vi "导出监测.vi"(4 "路径":path, 5 "错误常量":errorcluster caption="错误输入", 6 "报警信息":string[][](array[string]), 7 "计算数据":dbl[][](array[numeric]), 8 "监测名":string) -> (0 "错误常量 2":errorcluster caption="错误输出")   [LabVIEW 2018]
uses:
  <vilib>/Utility/file.llb/Write Delimited Spreadsheet (string).vi
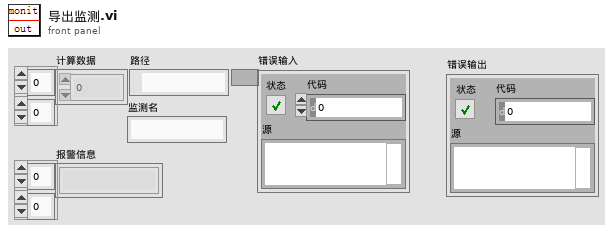
[diagram p1: front panel]
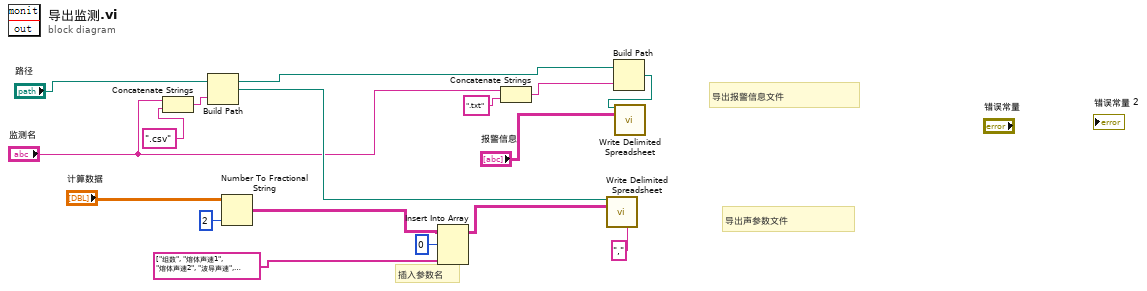
[diagram p0: block diagram]
diagram:
  # "导出声参数文件"
  # "导出报警信息文件"
  # "插入参数名"
  n1 = Concatenate Strings("监测名", ".csv" ("名称或相对路径")) -> (w14:string)
  n2 = Build Path(base path="路径", name or relative path=w14) -> (appended path=w16:path)
  n3 = Number To Fractional String(number="计算数据", precision (6)=i16 2 ("精度(6)")) -> (F-format string=w9:string[][])  [unwired: 2 in]
  n4 = Insert Into Array(array=w9, index (row)=0 ("索引 (行)"), new element=string[] ["组数", "熔体声速1", "熔体声速2", "波导声速", "声衰减系数", "声参量1  ", "声参量2  ", "x1", "x2     ", "x3", "x4       ", "y1", "y2", "y3", "y4"] ("新元素/子数组")) -> (w1:string[][])  [unwired: 1 in]
  n5 = Concatenate Strings("监测名", ".txt" ("字符串")) -> (w12:string)
  n6 = call-poly <vilib>:"Write Delimited Spreadsheet.vi"("file path (dialog if empty)"=w16, "2D data"=w1, "delimiter (\\t)"="," ("delimiter (\\t)")) -> ()  [unwired: 11 in, 2 out]
  n7 = Build Path(base path="路径", name or relative path=w12) -> (appended path=w13:path)
  n8 = call-poly <vilib>:"Write Delimited Spreadsheet.vi"("file path (dialog if empty)"=w13, "2D data"="报警信息") -> ()  [unwired: 12 in, 2 out]
